vi "IFNoise-Initialize.vi"(0 "Speaker":T5, 5 "State":T3, 7 "InvFilt Params":T4={"Min Frequency (Hz)"=1000.0, "Max Frequency (Hz)"=50000.0, "Length (points)"=1431000, "Sampling rate (Hz)"=100000.0, "Delay (ms)"=301.0, "Linear phase"=FALSE}, 9 "IFNoise-Params":T2={"Averages"=128, "Probe Mic Gain (dB)"=0.0, "Cal Mic Gain (dB)"=0.0, "Cal Mic Sens (dB V/SPL)"=0.0, "Attenuation (dB)"=20.0, "Sample size (s)"=128.0, "Input"=enum."Probe Mic"}, 11 "error in (no error)":errorcluster, 12 "Inverse Filter":bool) -> (3 "Max SPL":dbl, 4 "Runtime":T1, 15 "error out":errorcluster)   [LabVIEW 2015]
uses:
  <vilib>/Analysis/NI_AALPro.lvlib
  <vilib>/Analysis/5stat.llb/RMS (DBL).vi
  Utility VIs/Type Defs/Speaker ring.ctl
  Inverse Filter VIs/InvFilt-Params.ctl
  Cochlear Function Test Suite/LV Source/CFTS Main Panel SubVIs/CFTS-Experiment State.ctl
  Type Defs/IFNoise-Params.ctl
  Type Defs/IFNoise-Runtime.ctl
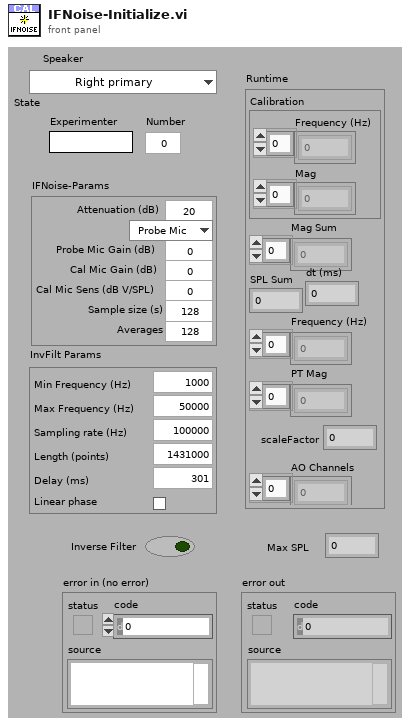
[diagram p1: front panel]
types:
  T1 = typedef "IFNoise-Runtime.ctl" = cluster{"Calibration":cluster{"Frequency (Hz)":dbl[], "Mag":dbl[]}, "Mag Sum":dbl[], "SPL Sum":dbl, "Frequency (Hz)":dbl[], "PT Mag":dbl[], "dt (ms)":dbl, "AO Channels":i32[], "scaleFactor":dbl}
  T2 = typedef "IFNoise-Params.ctl" = cluster{"Averages":i32, "Probe Mic Gain (dB)":dbl, "Cal Mic Gain (dB)":dbl, "Cal Mic Sens (dB V/SPL)":dbl, "Attenuation (dB)":dbl, "Sample size (s)":dbl, "Input":enum16{"Probe Mic", "Cal Mic", "Voltage Only"}}
  T3 = typedef "CFTS-Experiment State.ctl" = cluster{"Experimenter":string, "Number":u32, "Right":string, "Left":string, "Data Folder":path, "State File":path, "Version Info":string, "End Exposure Time":dbl, "Exposure Duration":string, "Run #":cluster{"CAP":i16, "ABR":i16, "DP":i16, "VsEP":i16, "MeasSeq":i16, "SubSeq":i16, "SFOAE":i16}}
  T4 = typedef "InvFilt-Params.ctl" = cluster{"Min Frequency (Hz)":dbl, "Max Frequency (Hz)":dbl, "Length (points)":i32, "Sampling rate (Hz)":dbl, "Delay (ms)":dbl, "Linear phase":bool}
  T5 = typedef "Speaker ring.ctl" = enum16{"Right primary", "Right secondary", "Left primary", "Left secondary"}
  T6 = cluster{"Interp Freq (Hz)":dbl[], "Magnitude (dB)":dbl[]}
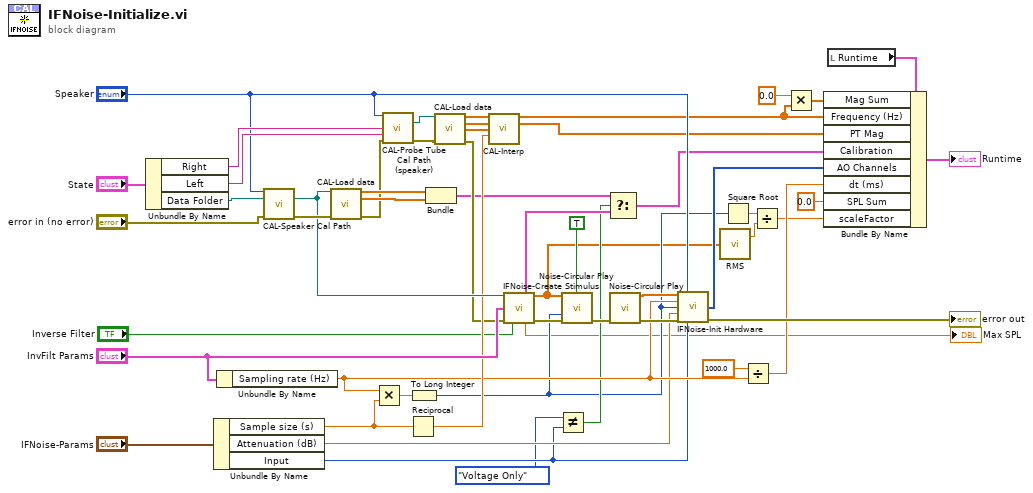
[diagram p0: block diagram]
diagram:
  n1 = Unbundle By Name("State") -> ("Right"=w49:string, "Left"=w48:string, "Data Folder"=w50:path)
  n2 = Unbundle By Name("IFNoise-Params") -> ("Sample size (s)"=w32:dbl, "Attenuation (dB)"=w24:dbl, "Input"=w10:enum16{"Probe Mic", "Cal Mic", "Voltage Only"})
  n3 = Unbundle By Name("InvFilt Params") -> ("Sampling rate (Hz)"=w25:dbl)
  n4 = call "CAL-Speaker Cal Path.vi"("Speaker"="Speaker", "Data Folder"=w50, "error in (no error)"="error in (no error)") -> ("Cal Path"=w35:path, "error out"=w37:errorcluster)  [unwired: 11 in]
  n5 = call "CAL-Load data.vi"("user path"=w35, "error in (no error)"=w37) -> ("Frequency (Hz)"=w47:dbl[], "Mag"=w46:dbl[], "error out"=w30:errorcluster)  [unwired: 6 in, 5 out]
  n6 = Multiply(x=w25, y=w32) -> (x*y=w39:dbl)
  n7 = call "CAL-Probe Tube Cal Path (speaker).vi"("Speaker"="Speaker", "Right"=w49, "Left"=w48, "error in (no error)"=w30) -> ("Probe Tube Cal Path"=w44:path, "error out"=w43:errorcluster)  [unwired: 10 in]
  n8 = Reciprocal(x=w32) -> (1/x=w31:dbl)
  n9 = To Long Integer(number=w39) -> (32bit integer=w5:i32)
  n10 = Bundle("Frequency (Hz)"=w47, "Mag"=w46) -> (w13:cluster{"Frequency (Hz)":dbl[], "Mag":dbl[]})  [unwired: 1 in]
  n11 = call "CAL-Load data.vi"("user path"=w44, "error in (no error)"=w43) -> ("Frequency (Hz)"=w42:dbl[], "Mag"=w41:dbl[], "Phase"=w40:dbl[], "error out"=w29:errorcluster)  [unwired: 6 in, 4 out]
  n12 = call "CAL-Interp.vi"("Frequency (Hz)"=w42, "Magnitude (dB)"=w41, "Phase (degrees)"=w40, "df (Hz)"=w31) -> ("Interp Freq (Hz)"=w17:dbl[], "Interp Magnitude (dB)"=w21:dbl[])  [unwired: 8 in, 2 out]
  n13 = call "IFNoise-Create Stimulus.vi"("Path"=w35, "InvFilt Params"="InvFilt Params", "error in (no error)"=w29, "Inverse Filter"="Inverse Filter") -> ("Mag Spec"=w11:T6, "Noise"=w3:dbl[], "Max SPL"=→"Max SPL":dbl, "error out"=w38:errorcluster)  [unwired: 8 in]
  n14 = Not Equal?(x=enum16{"Probe Mic", "Cal Mic", "Voltage Only"}."Voltage Only", y=w10) -> (x != y?=w9:bool)
  n15 = call "Noise-Circular Play.vi"("Noise (in)"=w3, "Init? (F)"=TRUE, "Npts"=w5, "error in (no error)"=w38) -> ("error out"=w33:errorcluster)  [unwired: 10 in, 1 out]
  n16 = Select(t=w13, s=w9, f=w11) -> (s? t:f=w12:T6)
  n17 = call "Noise-Circular Play.vi"("error in (no error)"=w33) -> ("Noise (out)"=w26:dbl[], "error out"=w28:errorcluster)  [unwired: 13 in]
  n18 = call "IFNoise-Init Hardware.vi"("AO Buffer"=w26, "Speaker"="Speaker", "Sampling rate (Hz)"=w25, "Npts"=w5, "Attenuation (dB)"=w24, "error in (no error)"=w28, "Input source"=w10) -> ("AO Channels"=w20:i32[], "error out"=→"error out":errorcluster)  [unwired: 7 in]
  n19 = call-poly <vilib>:"RMS.vi"("X"=w3) -> ("rms value"=w4:dbl)  [unwired: 1 out]
  n20 = Square Root(x=w5) -> (sqrt(x)=w6:dbl)
  n21 = Divide(x=1000.0, y=w25) -> (x/y=w19:dbl)
  n22 = Divide(x=w6, y=w4) -> (x/y=w7:dbl)
  n23 = Multiply(x=0.0, y=w17) -> (x*y=w16:dbl[])
  n24 = local read "Runtime"() -> (w22:T1)
  n25 = Bundle By Name(cluster=w22, "Mag Sum"=w16, "Frequency (Hz)"=w17, "PT Mag"=w21, "Calibration"=w12, "AO Channels"=w20, "dt (ms)"=w19, "SPL Sum"=0.0, "scaleFactor"=w7) -> (→"Runtime":T1)
